vi "Lost Array.vi"() -> (2 "Coloumn":i32[](array[numeric])=[30, 31, 32, 31, 29, 31, 33, 31, 28, 31, 34, 31, 27, 31, 35, 31, 26, 31, 36, 31, 25, 31, 37, 31, 24, 31, 38, 31, 23, 31, 39, 31, 22, 31, 40, 31, 21, 31, 41, 31, 20, 31, 42, 31, 19, 31, 43, 31, 18, 31, 44, 31, 17, 31, 45, 31, 16, 31, 46, 31], 3 "Row":i32[](array[numeric])=[31, 30, 31, 32, 31, 29, 31, 33, 31, 28, 31, 34, 31, 27, 31, 35, 31, 26, 31, 36, 31, 25, 31, 37, 31, 24, 31, 38, 31, 23, 31, 39, 31, 22, 31, 40, 31, 21, 31, 41, 31, 20, 31, 42, 31, 19, 31, 43, 31, 18, 31, 44, 31, 17, 31, 45, 31, 16, 31, 46])   [LabVIEW 2016]
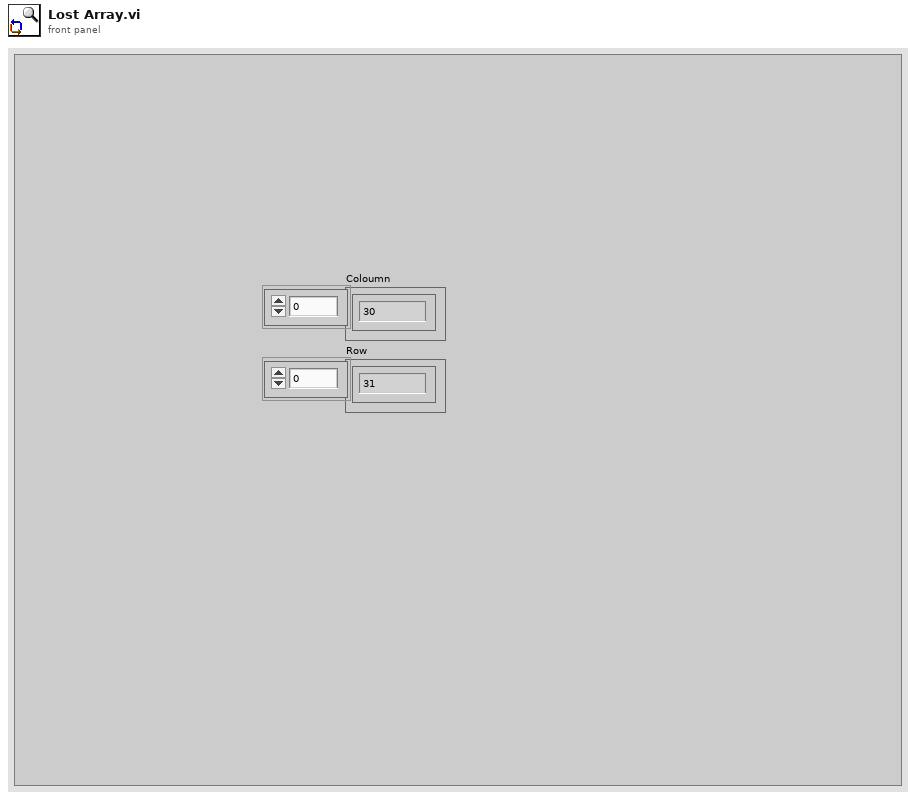
[diagram p1: front panel]
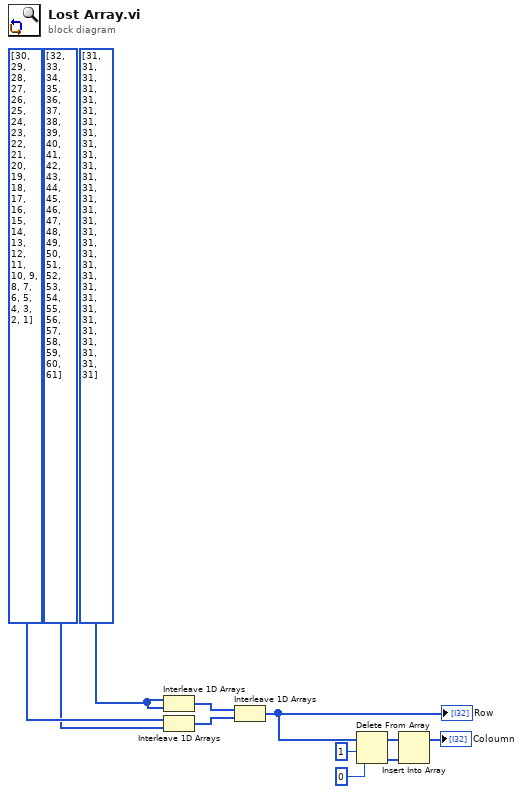
[diagram p0: block diagram]
diagram:
  w11 = i32[] [31, 31, 31, 31, 31, 31, 31, 31, 31, 31, 31, 31, 31, 31, 31, 31, 31, 31, 31, 31, 31, 31, 31, 31, 31, 31, 31, 31, 31, 31]
  n1 = Interleave 1D Arrays(w11, w11) -> (w8:i32[])
  n2 = Interleave 1D Arrays(i32[] [30, 29, 28, 27, 26, 25, 24, 23, 22, 21, 20, 19, 18, 17, 16, 15, 14, 13, 12, 11, 10, 9, 8, 7, 6, 5, 4, 3, 2, 1], i32[] [32, 33, 34, 35, 36, 37, 38, 39, 40, 41, 42, 43, 44, 45, 46, 47, 48, 49, 50, 51, 52, 53, 54, 55, 56, 57, 58, 59, 60, 61]) -> (w7:i32[])
  n3 = Interleave 1D Arrays(w8, w7) -> (w2:i32[])
  "Row" <- w2
  n4 = Delete From Array(array=w2, length=1, index=0) -> (deleted portion=w4:i32[], array with subset deleted=w3:i32[])
  n5 = Insert Into Array(array=w3, new element=w4) -> (→"Coloumn":i32[])  [unwired: 1 in]
